vi "Update OneOf Field Accessor.vi"(8 "error in (no error)":errorcluster, 9 "message element metadata":T1={"Field Name"="nested_message_2", "Embedded Message Name"="echo_array_NestedMessage2", "Protobuf Index"=3, "MessageElementType"=enum."MessageValue", "Repeated"=FALSE, "Is in Oneof"=TRUE, "Oneof Container Name"="echo_array_NestedMessage_union"}, 10 "class in":refnum<vi>, 11 "library in":refnum<vi>) -> (0 "error out":errorcluster, 2 "class out":refnum<vi>, 3 "library out":refnum<vi>)   [LabVIEW 2019, in "gRPC Template Creation Utility.lvlib"]
uses:
  gRPC Template Creation Utility.lvlib
  TypeDefs/Message Element Type.ctl
  TypeDefs/Message Element Metadata (Scripting).ctl
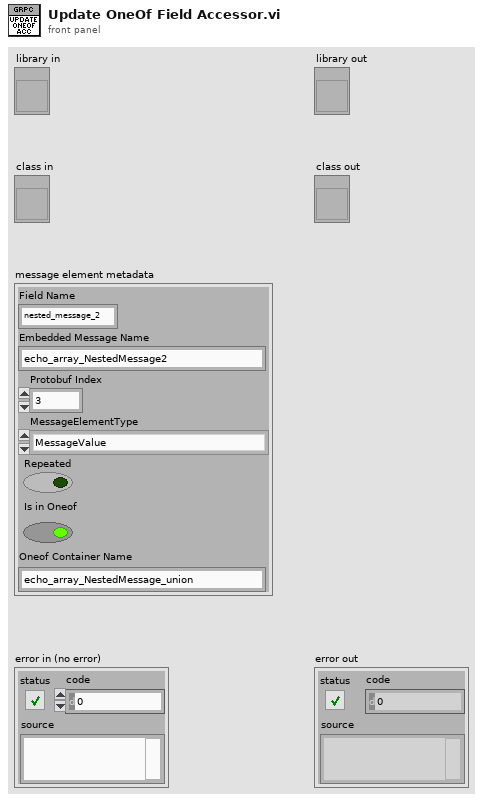
[diagram p1: front panel]
types:
  T1 = typedef "gRPC Template Creation Utility.lvlib/Message Element Metadata (Scripting).ctl" = cluster{"Field Name":string, "Embedded Message Name":string, "Protobuf Index":i32, "MessageElementType":T2, "Repeated":bool, "Is in Oneof":bool, "Oneof Container Name":string}
  T2 = typedef "gRPC Template Creation Utility.lvlib/Message Element Type.ctl" = enum32{"Int32Value", "FloatValue", "DoubleValue", "BoolValue", "StringValue", "MessageValue", "Int64Value", "UInt32Value", "UInt64Value", "EnumValue", "Bytes", "Fixed64", "Fixed32", "SFixed64", "SFixed32", "SInt64", "SInt32"}
  T3 = typedef "grpc-lvsupport-release.lvlib/Well Known Types.ctl" = enum32{"None", "Double2DArray", "String2DArray"}
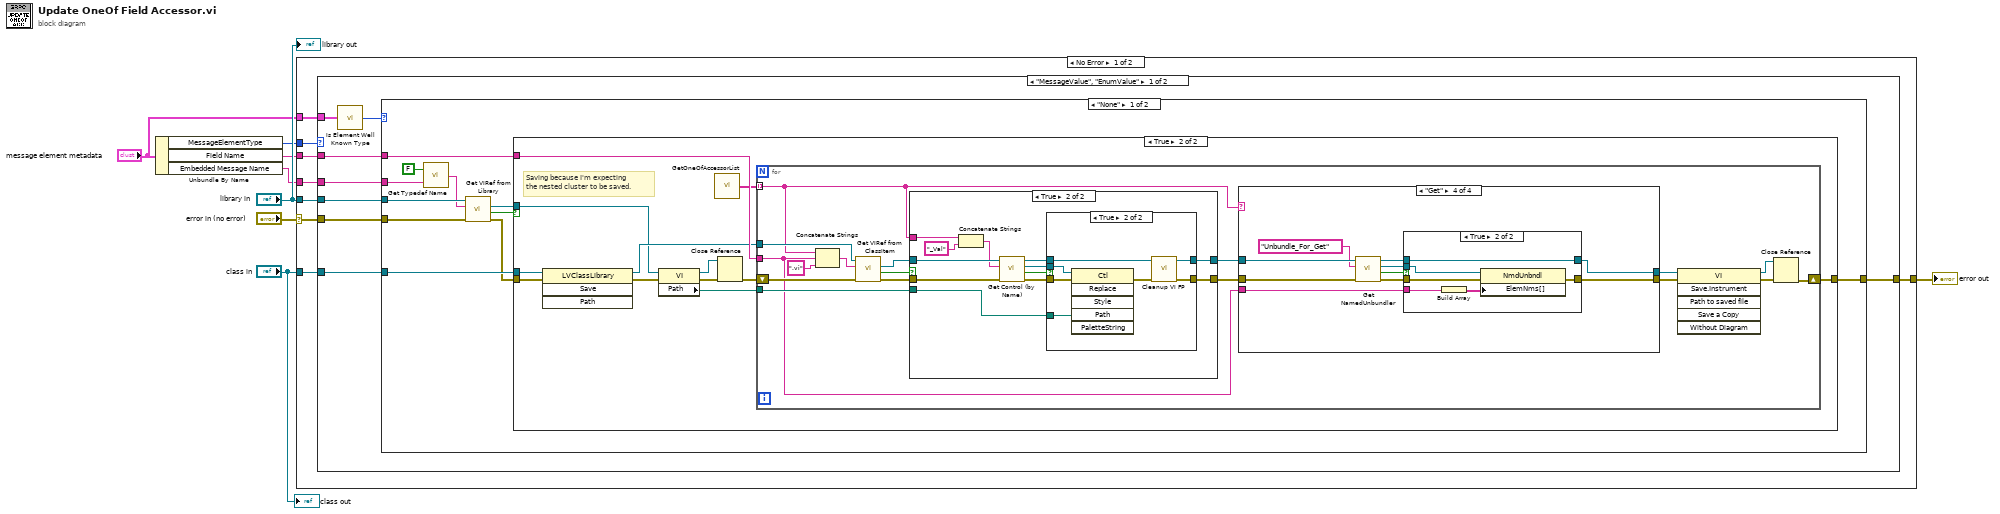
[diagram p0: block diagram]
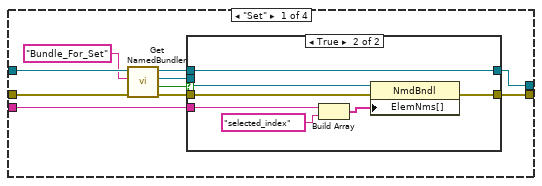
[diagram p3: hidden frame]
diagram:
  n1 = Unbundle By Name("message element metadata") -> ("MessageElementType"=w4:T2, "Field Name"=w3:string, "Embedded Message Name"=w2:string)
  n2 = case shown="No Error" "error in (no error)" {
    selector: "error in (no error)" -> [w10 w132]
    tunnel: [w16 w132] -> w8
    tunnel: w2 -> [w15 _]
    tunnel: w3 -> [w14 _]
    tunnel: "library in" -> [w13 _]
    tunnel: w4 -> [w12 _]
    tunnel: "class in" -> [w11 _]
    tunnel: "message element metadata" -> [w9 _]
    frame No Error {
      n3 = case shown="\"MessageValue\", \"EnumValue\"" w12 {
        tunnel: w10 -> [w20 w131]
        tunnel: w11 -> [w24 _]
        tunnel: w13 -> [w21 _]
        tunnel: w14 -> [w23 _]
        tunnel: w15 -> [w22 _]
        tunnel: [w19 w131] -> w16
        tunnel: w9 -> [w18 _]
        frame "MessageValue", "EnumValue" {
          n4 = call "Is Element Well Known Type.vi"("element metadata"=w18) -> ("well known type"=w17:T3)
          n5 = case shown="\"None\"" w17 {
            tunnel: w24 -> [w35 _]
            tunnel: w23 -> [w34 _]
            tunnel: w22 -> [w33 _]
            tunnel: w21 -> [w32 _]
            tunnel: w20 -> [w30 w130]
            tunnel: [w25 w130] -> w19
            frame "None" {
              n6 = call "Get Typedef Name.vi"("embedded message name"=w33, "generate serialization helpers"=FALSE ("Generate_SerializationHelper")) -> ("typedef name"=w31:string)
              n7 = call "Get VIRef from Library.vi"("error in (no error)"=w30, "item name"=w31, "library in"=w32) -> ("error out"=w29:errorcluster, "found"=w28:bool, "vi"=w27:refnum<vi>)  [unwired: 5 in, 1 out]
              n8 = case shown="True" w28 {
                tunnel: w34 -> [_ w48]
                tunnel: w35 -> [_ w46]
                tunnel: w29 -> [w36 w44]
                tunnel: [w36 w40] -> w25
                tunnel: w27 -> [_ w43]
                frame False {
                }
                frame True {
                  # "Saving because I'm expecting\nthe nested cluster to be saved."
                  n9 = invoke class="LVClassLibrary" method="Save"(reference=w46, error in=w44) -> (reference out=w45:refnum<vi>, error out=w41:errorcluster)  [unwired: 2 in, 2 out]
                  n10 = property class="VI"(reference=w43, error in=w41) -> (reference out=w38:refnum<vi>, error out=w39:errorcluster, "Path"=w42:path)
                  n11 = call "GetOneOfAccessorList.vi"() -> ("Array"=w47:string[])
                  n12 = Close Reference(reference=w38, error in (no error)=w39) -> (error out=w37:errorcluster)
                  n13 = for {
                    tunnel: w47 -> [w55] mode=indexing
                    tunnel: w48 -> [w54]
                    tunnel: w45 -> [w64]
                    tunnel: w42 -> [w60]
                    shift-right: [w49] -> w40
                    shift-left: w37 -> [w58]
                    n14 = Concatenate Strings(w55, w54, ".vi" ("string")) -> (w63:string)
                    n15 = call "Get VIRef from ClassItem.vi"("error in (no error)"=w58, "item name"=w63, "class in"=w64) -> ("error out"=w59:errorcluster, "found"=w62:bool, "vi"=w61:refnum<vi>)  [unwired: 5 in, 1 out]
                    n16 = case shown="True" w62 {
                      tunnel: w61 -> [w108 w118]
                      tunnel: w55 -> [_ w119]
                      tunnel: w60 -> [_ w115]
                      tunnel: w59 -> [w107 w113]
                      tunnel: [w108 w109] -> w57
                      tunnel: [w107 w111] -> w56
                      frame False {
                      }
                      frame True {
                        n17 = Concatenate Strings(w119, "_Val" ("string")) -> (w112:string)
                        n18 = call "Get Control (by Name).vi"("error in (no error)"=w113, "Control Label"=w112, "Owner VI in"=w118) -> ("error out"=w114:errorcluster, "Found ?"=w117:bool, "Control Refnum"=w116:refnum<vi>, "Owner VI out"=w110:refnum<vi>)  [unwired: 5 in]
                        n19 = case shown="True" w117 {
                          tunnel: w116 -> [_ w129]
                          tunnel: w115 -> [_ w128]
                          tunnel: w114 -> [w122 w127]
                          tunnel: [w122 w125] -> w111
                          tunnel: w110 -> [w121 w124]
                          tunnel: [w121 w123] -> w109
                          frame False {
                            # "This will not be found for Has<Field>.vi"
                          }
                          frame True {
                            n20 = invoke class="Ctl" method="Replace"(reference=w129, error in=w127, "Path"=w128) -> (error out=w126:errorcluster)  [unwired: 3 in, 5 out]
                            n21 = call "Cleanup VI FP.vi"("error in"=w126, "vi in"=w124) -> ("error out"=w125:errorcluster, "vi out"=w123:refnum<vi>)  [unwired: 8 in]
                          }
                        }
                      }
                    }
                    n22 = case shown="\"Get\"" w55 {
                      tunnel: w57 -> [w75 w85 w87 w98]
                      tunnel: w56 -> [w73 w86 w88 w96]
                      tunnel: w54 -> [w70 _ _ w93]
                      tunnel: [w68 w86 w88 w91] -> w53
                      tunnel: [w66 w85 w87 w89] -> w52
                      frame "Set" {
                        n23 = call "Get NamedBundler.vi"("error in (no error)"=w73, "Label"="Bundle_For_Set", "Owner VI in"=w75) -> ("error out"=w69:errorcluster, "Found ?"=w72:bool, "NamedBundler ref out"=w71:refnum<vi>, "Owner VI out"=w67:refnum<vi>)  [unwired: 5 in]
                        n24 = case shown="True" w72 {
                          tunnel: w71 -> [_ w84]
                          tunnel: w70 -> [_ w82]
                          tunnel: w69 -> [w77 w80]
                          tunnel: [w77 w79] -> w68
                          tunnel: w67 -> [w76 w78]
                          tunnel: [w76 w78] -> w66
                          frame False {
                          }
                          frame True {
                            n25 = Build Array(w82, "selected_index" ("element")) -> (w83:string[])
                            n26 = property class="NmdBndl"(reference=w84, error in=w80, "ElemNms[]"=w83) -> (error out=w79:errorcluster)  [unwired: 1 out]
                          }
                        }
                      }
                      frame "Has" {
                      }
                      frame Default {
                      }
                      frame "Get" {
                        n27 = call "Get NamedUnbundler.vi"("error in (no error)"=w96, "Label"="Unbundle_For_Get", "Owner VI in"=w98) -> ("error out"=w92:errorcluster, "Found ?"=w95:bool, "NamedUnbundler ref out"=w94:refnum<vi>, "Owner VI out"=w90:refnum<vi>)  [unwired: 5 in]
                        n28 = case shown="True" w95 {
                          tunnel: w94 -> [_ w106]
                          tunnel: w93 -> [_ w104]
                          tunnel: w92 -> [w100 w103]
                          tunnel: [w100 w102] -> w91
                          tunnel: w90 -> [w99 w101]
                          tunnel: [w99 w101] -> w89
                          frame False {
                          }
                          frame True {
                            n29 = Build Array(w104) -> (w105:string[])
                            n30 = property class="NmdUnbndl"(reference=w106, error in=w103, "ElemNms[]"=w105) -> (error out=w102:errorcluster)  [unwired: 1 out]
                          }
                        }
                      }
                    }
                    n31 = invoke class="VI" method="Save.Instrument"(reference=w52, error in=w53) -> (reference out=w50:refnum<vi>, error out=w51:errorcluster)  [unwired: 4 in, 4 out]
                    n32 = Close Reference(reference=w50, error in (no error)=w51) -> (error out=w49:errorcluster)
                  }
                }
              }
            }
            frame Default {
            }
          }
        }
        frame Default {
        }
      }
    }
    frame Error {
    }
  }
  "error out" <- w8
  "library out" <- "library in"
  "class out" <- "class in"
